vi "get stream specifications.vi"(8 "error in":errorcluster, 11 "module configuration in":refnum<class "TBM module configuration.lvclass">) -> (0 "error out":errorcluster, 1 "subscribers":T1[](array[typedef]), 2 "publishers":T1[](array[typedef]), 3 "module configuration out":refnum<class "TBM module configuration.lvclass">)   [LabVIEW 2013, in "TBM module configuration.lvclass"]
uses:
  TBM module configuration.lvclass
  stream specification.ctl
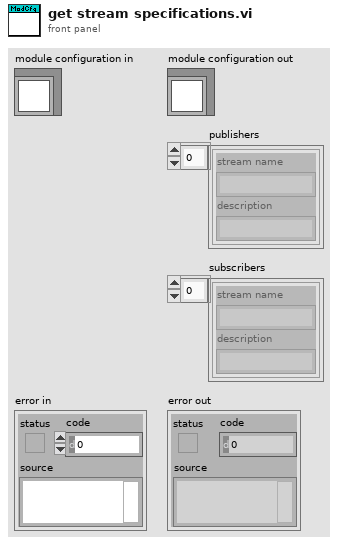
[diagram p1: front panel]
types:
  T1 = typedef "TBM module configuration.lvclass/stream specification.ctl" = cluster{"stream name":string, "description":string}
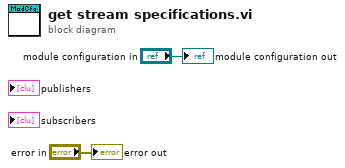
[diagram p0: block diagram]
diagram:
  "error out" <- "error in"
  "module configuration out" <- "module configuration in"
